vi "ExFileReadNConvertToDatatype.vi"() -> ()   [LabVIEW 2010]
panel:
  in  "Output file name":path=path "C:/Program Files/SIToolKit/LabVIEW/Data Files/test"
  in  "data type":u32=7 min=1 max=8 step=1
  in  "Full File Name":path=path "C:/Program Files/SIToolKit/LabVIEW/Data Files/Color.SPE"
  in  "?":bool
  in  "FileType":u32=67371008
  out "error out":errorcluster
  in  "error in (no error)":errorcluster
  # "ExReadFileNconvertToDatatype.vi\nThis example will read in a file of the\nselected data type and display as datatype frame.\nWhen finished viewing data, make sure to\nuse the STOP button to close the display."
  # "File Types:\nSPE = 67371008\nTIF   = 67174400\nPMI  = 67436544"
  # "Browse match pattern is set to *.spe.  Modify this if different file type is needed."
  # "This will properly close\nthe image and\ndeallocate memory."
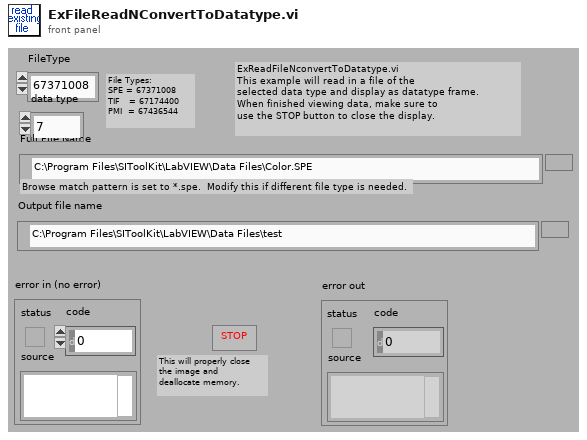
[diagram p1: front panel]
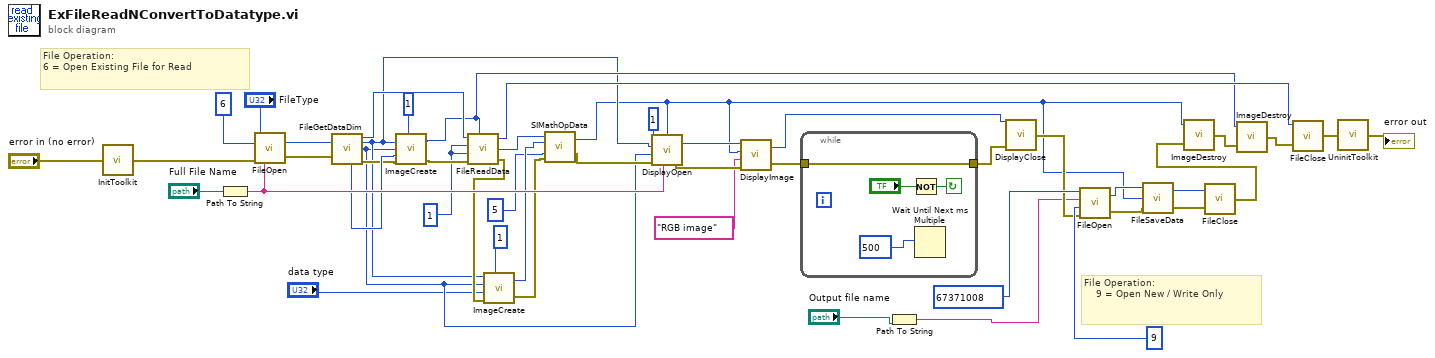
[diagram p0: block diagram]
diagram:
  w34 = 1
  # "File Operation:\n    9 = Open New / Write Only"
  # "File Operation:\n6 = Open Existing File for Read"
  n1 = call <userlib>:"InitToolkit.vi"("error in"="error in (no error)") -> ("error out"=w46:errorcluster)
  n2 = Path To String(path="Full File Name") -> (string=w37:string)
  n3 = call <userlib>:"FileOpen.vi"("error in"=w46, "File Operations"=u32 6 ("File Operation"), "FileName"=w37, "File Type"="FileType") -> ("error out"=w44:errorcluster, "File Handle"=w43:u32)
  n4 = call <userlib>:"FileGetDataDim.vi"("File Handle"=w43, "error in"=w44) -> ("Data Type"=w24:u32, "File Handle"=w36:u32, "X dim"=w6:u32, "Y dim"=w5:u32, "error out"=w21:errorcluster)  [unwired: 1 out]
  n5 = call <userlib>:"ImageCreate.vi"("X dimension"=w6, "Y dimension"=w5, "Data Type"=w24, "error in"=w21, "Number Of Frames"=1) -> ("Image Handle"=w26:u32, "error out"=w35:errorcluster)
  n6 = call <userlib>:"FileReadData.vi"("File Handle"=w36, "Start Frame"=w34, "End Frame"=w34, "error in"=w35, "Image Handle"=w26) -> ("File Handle"=w33:u32, "Image Handle"=w18:u32, "error out"=w22:errorcluster)
  n7 = call <userlib>:"ImageCreate.vi"("X dimension"=w6, "Y dimension"=w5, "Data Type"="data type", "error in"=w22, "Number Of Frames"=1) -> ("Image Handle"=w19:u32, "error out"=w20:errorcluster)
  n8 = call <userlib>:"SIMathOpData.vi"("error in (no error)"=w20, "Operation"=5, "Result Handle"=w19, "Data Handle"=w18) -> ("error out"=w16:errorcluster, "Result Handle"=w4:u32)
  n9 = call <userlib>:"DisplayOpen.vi"("Display Title"=w37, "Image Handle"=w4, "error in"=w16, "Display Height"=w5, "Display Width"=w6, "Display Type"=1) -> ("error out"=w32:errorcluster, "Display Handle"=w31:u32)
  n10 = call <userlib>:"DisplayImage.vi"("error in"=w32, "Title"="RGB image", "Image Handle"=w4, "Display Handle"=w31) -> ("error out"=w25:errorcluster, "Display Handle"=w30:u32)
  n11 = while {
    tunnel: w25 -> [w49]
    tunnel: [w49] -> w9
    stop <- w51 continue-if-true
    n12 = Not(x="?") -> (.not. x?=w51:bool)
    n13 = Wait Until Next ms Multiple(millisecond multiple=500) -> ()  [unwired: 1 out]
  }
  n14 = Path To String(path="Output file name") -> (string=w1:string)
  n15 = call <userlib>:"DisplayClose.vi"("error in"=w9, "Display Handle"=w30) -> ("error out"=w8:errorcluster)
  n16 = call <userlib>:"FileOpen.vi"("error in"=w8, "File Operations"=9, "FileName"=w1, "File Type"=67371008) -> ("error out"=w15:errorcluster, "File Handle"=w13:u32)
  n17 = call <userlib>:"FileSaveData.vi"("error in"=w15, "Image Handle"=w4, "File Handle"=w13) -> ("error out"=w14:errorcluster, "File Handle"=w12:u32)
  n18 = call <userlib>:"FileClose.vi"("error in"=w14, "File Handle"=w12) -> ("error out"=w7:errorcluster)
  n19 = call <userlib>:"ImageDestroy.vi"("error in"=w7, "Data handle"=w4) -> ("error out"=w29:errorcluster)
  n20 = call <userlib>:"ImageDestroy.vi"("error in"=w29, "Data handle"=w26) -> ("error out"=w28:errorcluster)
  n21 = call <userlib>:"FileClose.vi"("error in"=w28, "File Handle"=w33) -> ("error out"=w40:errorcluster)
  n22 = call <userlib>:"UninitToolkit.vi"("error in"=w40) -> ("error out"=→"error out":errorcluster)
